vi "Add AO Register - Right Click.vi"(11 "Node Ptr":T1 format="%.0x") -> ()   [LabVIEW 2020, in "Modbus Master System Explorer.lvlib"]
uses:
  Modbus Master System Explorer.lvlib
  <vilib>/NI VeriStand/Custom Device API/Custom Device Item Ref.ctl
  <vilib>/NI VeriStand/Custom Device Tools/Custom Device Utility Library/Custom Device Utility Library.lvlib
  <vilib>/NI VeriStand/Custom Device API/Custom Device API.lvlib
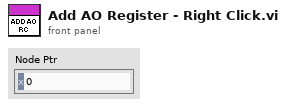
[diagram p1: front panel]
types:
  T1 = typedef "Custom Device API.lvlib/Custom Device Item Ref.ctl" = u64
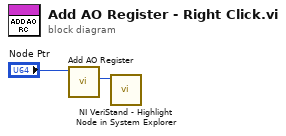
[diagram p0: block diagram]
diagram:
  n1 = call "Add AO Register.vi"("Node Ref In"="Node Ptr") -> ("Channel Ref out"=w1:T1)  [unwired: 8 in, 2 out]
  n2 = call <vilib>:"NI VeriStand - Highlight Node in System Explorer.vi"("Item Ref in"=w1) -> ()  [unwired: 9 in, 2 out]
